vi "StitchTestHeight.vi"() -> ()   [LabVIEW 2014]
panel:
  in  "SaveRaw":bool
  out "Intensity Graph":u32[][](graph)
  out "Yind":i32[](array[numeric])
  out "Xind":i32[](array[numeric])
  out "filenames":string[](array[string])
  in  "PathToVK4":path
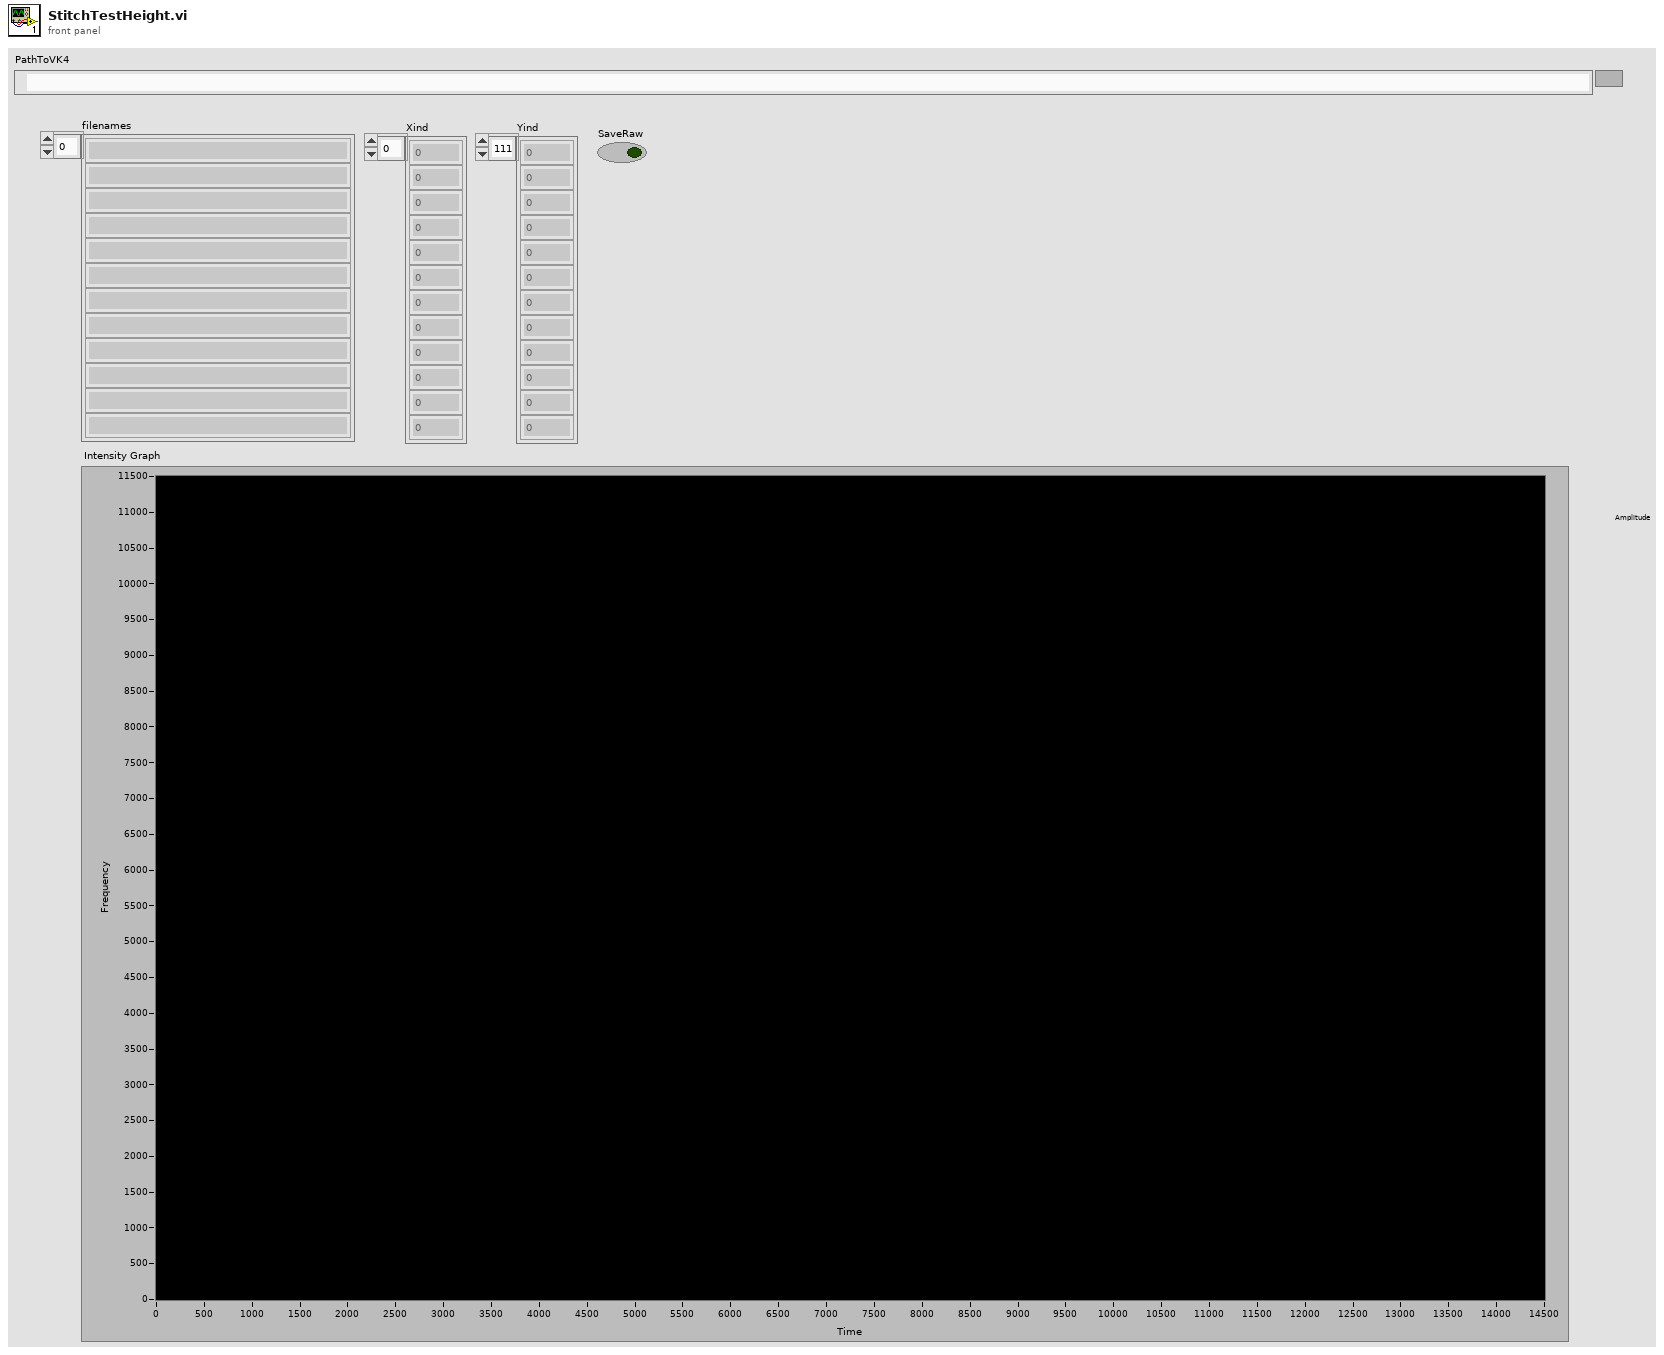
[diagram p1: front panel]
types:
  T1 = cluster{"left":i16, "top":i16, "right":i16, "bottom":i16}
  T2 = enum16{"big-endian, network order", "native, host order", "little-endian"}
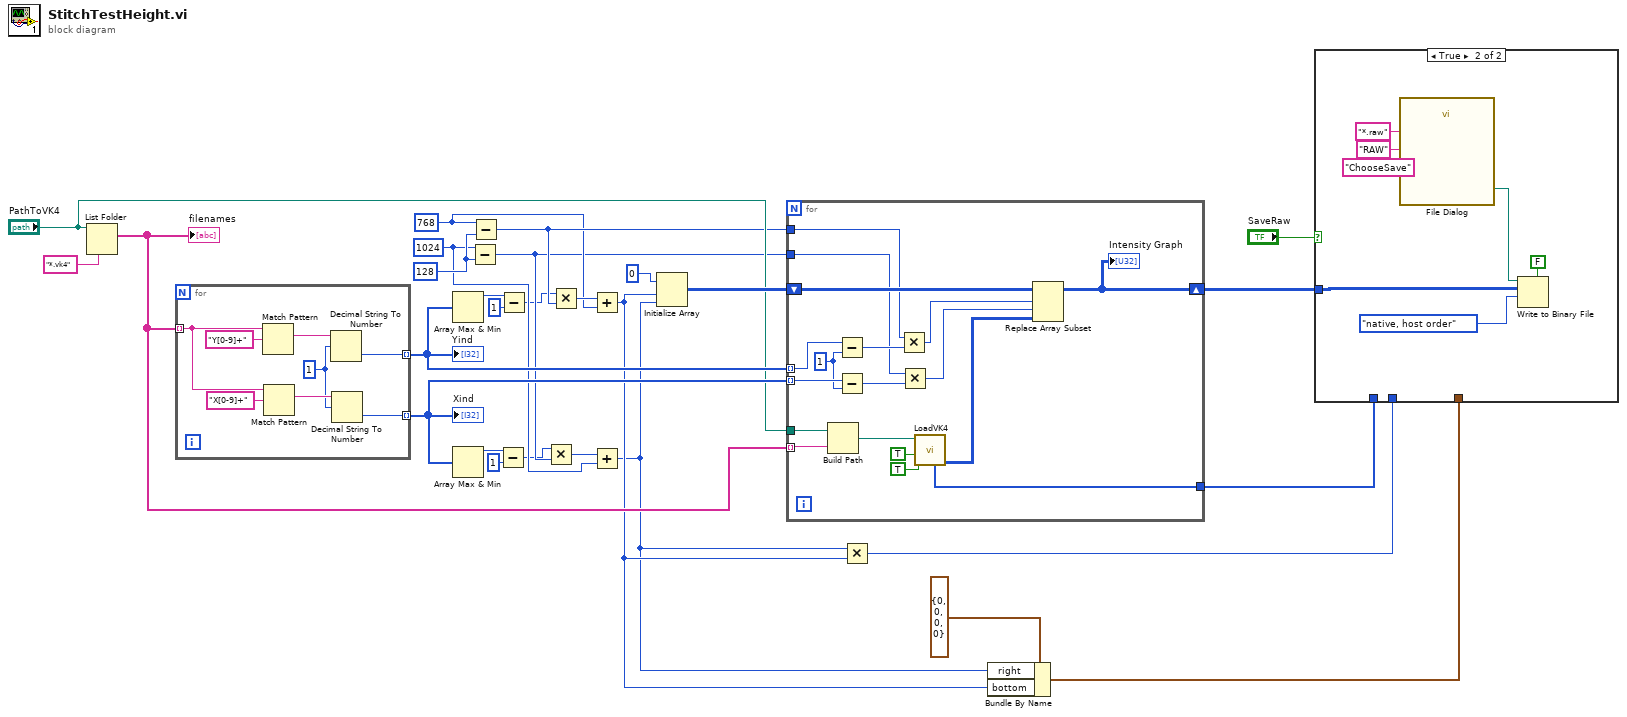
[diagram p0: block diagram]
diagram:
  w17 = 768
  w20 = 128 ("y")
  w16 = 1024
  n1 = List Folder(path="PathToVK4", pattern="*.vk4") -> (filenames=w25:string[])  [unwired: 2 in, 3 out]
  "filenames" <- w25
  n2 = for {
    tunnel: w25 -> [w32] mode=indexing
    tunnel: [w30] -> w23 mode=indexing
    tunnel: [w29] -> w22 mode=indexing
    w31 = 1 ("offset")
    n3 = Match Pattern(string=w32, regular expression="Y[0-9]+") -> (match substring=w35:string)  [unwired: 1 in, 3 out]
    n4 = Match Pattern(string=w32, regular expression="X[0-9]+") -> (match substring=w34:string)  [unwired: 1 in, 3 out]
    n5 = Decimal String To Number(string=w35, offset=w31) -> (number=w30:i32)  [unwired: 1 in, 1 out]
    n6 = Decimal String To Number(string=w34, offset=w31) -> (number=w29:i32)  [unwired: 1 in, 1 out]
  }
  "Xind" <- w22
  "Yind" <- w23
  n7 = Array Max & Min(array=w23) -> (max value=w6:i32)  [unwired: 3 out]
  n8 = Array Max & Min(array=w22) -> (max value=w2:i32)  [unwired: 3 out]
  n9 = Subtract(x=w16, y=w20) -> (x-y=w15:i32)
  n10 = Subtract(x=w17, y=w20) -> (x-y=w18:i32)
  n11 = Subtract(x=w2, y=1) -> (x-y=w1:i32)
  n12 = Subtract(x=w6, y=1) -> (x-y=w5:i32)
  n13 = Multiply(x=w1, y=w15) -> (x*y=w27:i32)
  n14 = Multiply(x=w5, y=w18) -> (x*y=w28:i32)
  n15 = Add(x=w28, y=w17) -> (x+y=w8:i32)
  n16 = Add(x=w27, y=w16) -> (x+y=w7:i32)
  n17 = Initialize Array(u32 0, w8, w7) -> (w24:u32[][])
  n18 = for {
    tunnel: w25 -> [w54] mode=indexing
    tunnel: "PathToVK4" -> [w53]
    tunnel: w23 -> [w49] mode=indexing
    tunnel: w22 -> [w48] mode=indexing
    tunnel: w15 -> [w39]
    shift-right: [w43] -> w14
    shift-left: w24 -> [w44]
    tunnel: w18 -> [w40]
    tunnel: [w38] -> w13
    w47 = 1 ("y")
    n19 = Build Path(base path=w53, name or relative path=w54) -> (appended path=w52:path)
    n20 = Subtract(x=w49, y=w47) -> (x-y=w46:i32)
    n21 = Subtract(x=w48, y=w47) -> (x-y=w45:i32)
    n22 = Multiply(x=w40, y=w46) -> (x*y=w41:i32)
    n23 = Multiply(x=w39, y=w45) -> (x*y=w42:i32)
    n24 = call "LoadVK4.vi"("SaveRaw"=TRUE, "SavePics"=TRUE, "PathToVK4"=w52) -> ("HeightArray"=w37:u32[][], "IntenLU"=w38:u32[])  [unwired: 4 in, 3 out]
    n25 = Replace Array Subset(array=w44, new element=w37, index (row)=w41, index (col)=w42) -> (w43:u32[][])
    "Intensity Graph" <- w43
  }
  n26 = Multiply(x=w7, y=w8) -> (x*y=w11:i32)
  n27 = Bundle By Name(cluster=T1 {"left"=0, "top"=0, "right"=0, "bottom"=0} ("Rectangle"), "right"=w7, "bottom"=w8) -> (w9:T1)
  n28 = case shown="True" "SaveRaw" {
    tunnel: w14 -> [_ w58]
    tunnel: w13 -> [_ _]
    tunnel: w11 -> [_ _]
    tunnel: w9 -> [_ _]
    frame False {
    }
    frame True {
      n29 = call "File Dialog"("prompt"="ChooseSave", "pattern (all files)"="*.raw", "pattern label"="RAW") -> ("selected path"=w56:path)  [unwired: 9 in, 3 out]
      n30 = Write to Binary File(file (use dialog)=w56, data=w58, 5:FALSE ("prepend array or string size? (T)"), 9:T2."native, host order" ("byte order (0:big-endian, network order)")) -> ()  [unwired: 2 in, 3 out]
    }
  }
